vi "bats.parser.hostToFpga.testRunner.vi"(9 "Test.Messages":variant[](array[variant]), 10 "Expected OrderBook.Command[]":T1[](array[typedef]), 11 "Test.MessagesOld":T3[](array[typedef])) -> (0 "Failures.Count":i32=1, 2 "Passed":bool, 3 "OrderBook.Command[]":T1[](array[typedef]), 4 "Debug":u64[](array[numeric]) format="%.0x")   [LabVIEW 2020]
uses:
  <vilib>/rvi/interface/nirviOpenFPGA/nirviOpenFPGA.xnode
  <vilib>/rvi/interface/nirviMethod/nirviMethod.xnode
  <vilib>/rvi/interface/nirviCloseFPGA/nirviCloseFPGA.xnode
  <vilib>/rvi/errors/niLvFpgaMergeErrorWithErrorCode.vi
  <vilib>/FPGAPlugInAG/Dynamic/niLvFpga_ReadFifo_Dynamic.vi
  <vilib>/rvi/interface/nirviReadWriteControl/nirviReadWriteControl.xnode
  <vilib>/rvi/interface/Simulation/niFpgaSimulationCallBeginRW.vi
  <vilib>/rvi/errors/niLvFpgaAdjustHostInterfaceError.vi
  builds/fpganow.common/fpganow.common.host.lvlib
  NiFpgaLv.dll
  <vilib>/Utility/error.llb/Error Cluster From Error Code.vi
  fpga/bats.parser.test.vi
  <vilib>/FPGAPlugInAG/Dynamic/niLvFpga_WriteFifo_Dynamic.vi
  <vilib>/FPGAPlugInAG/Dynamic/niLvFpga_Close_Dynamic.vi
  pitch/oldMessageType.ctl
  pitch/SequencedUnitHeader/SequencedUnitHeader.Parameters.ctl
  pitch/SequencedUnitHeader/SequencedUnitHeader.lvclass
  Message.Spec.ctl
  pitch/Time/Time.Parameters.ctl
  pitch/Time/Time.lvclass
  pitch/AddOrder/AddOrderLong.Parameters.ctl
  pitch/AddOrder/AddOrderLong.lvclass
  pitch/ModifyOrder/ModifyOrderLong.Parameters.ctl
  pitch/ModifyOrder/ModifyOrderLong.lvclass
  builds/fpganow.common/orderbook.command.ctl
  builds/fpganow.common/fpganow.common.fpga.lvlib
  builds/fpganow.common/orderbook.command.type.ctl
panel:
  out "size(s)":i32
  out "Words.Out":u16[](array[numeric]) format="%.0x"
  out "Data.size":i32=16
  in  "Execute?":bool=TRUE
  out "Data":u64[](array[numeric]) format="%.0x"
  out "error out":errorcluster
  in  "error in":errorcluster
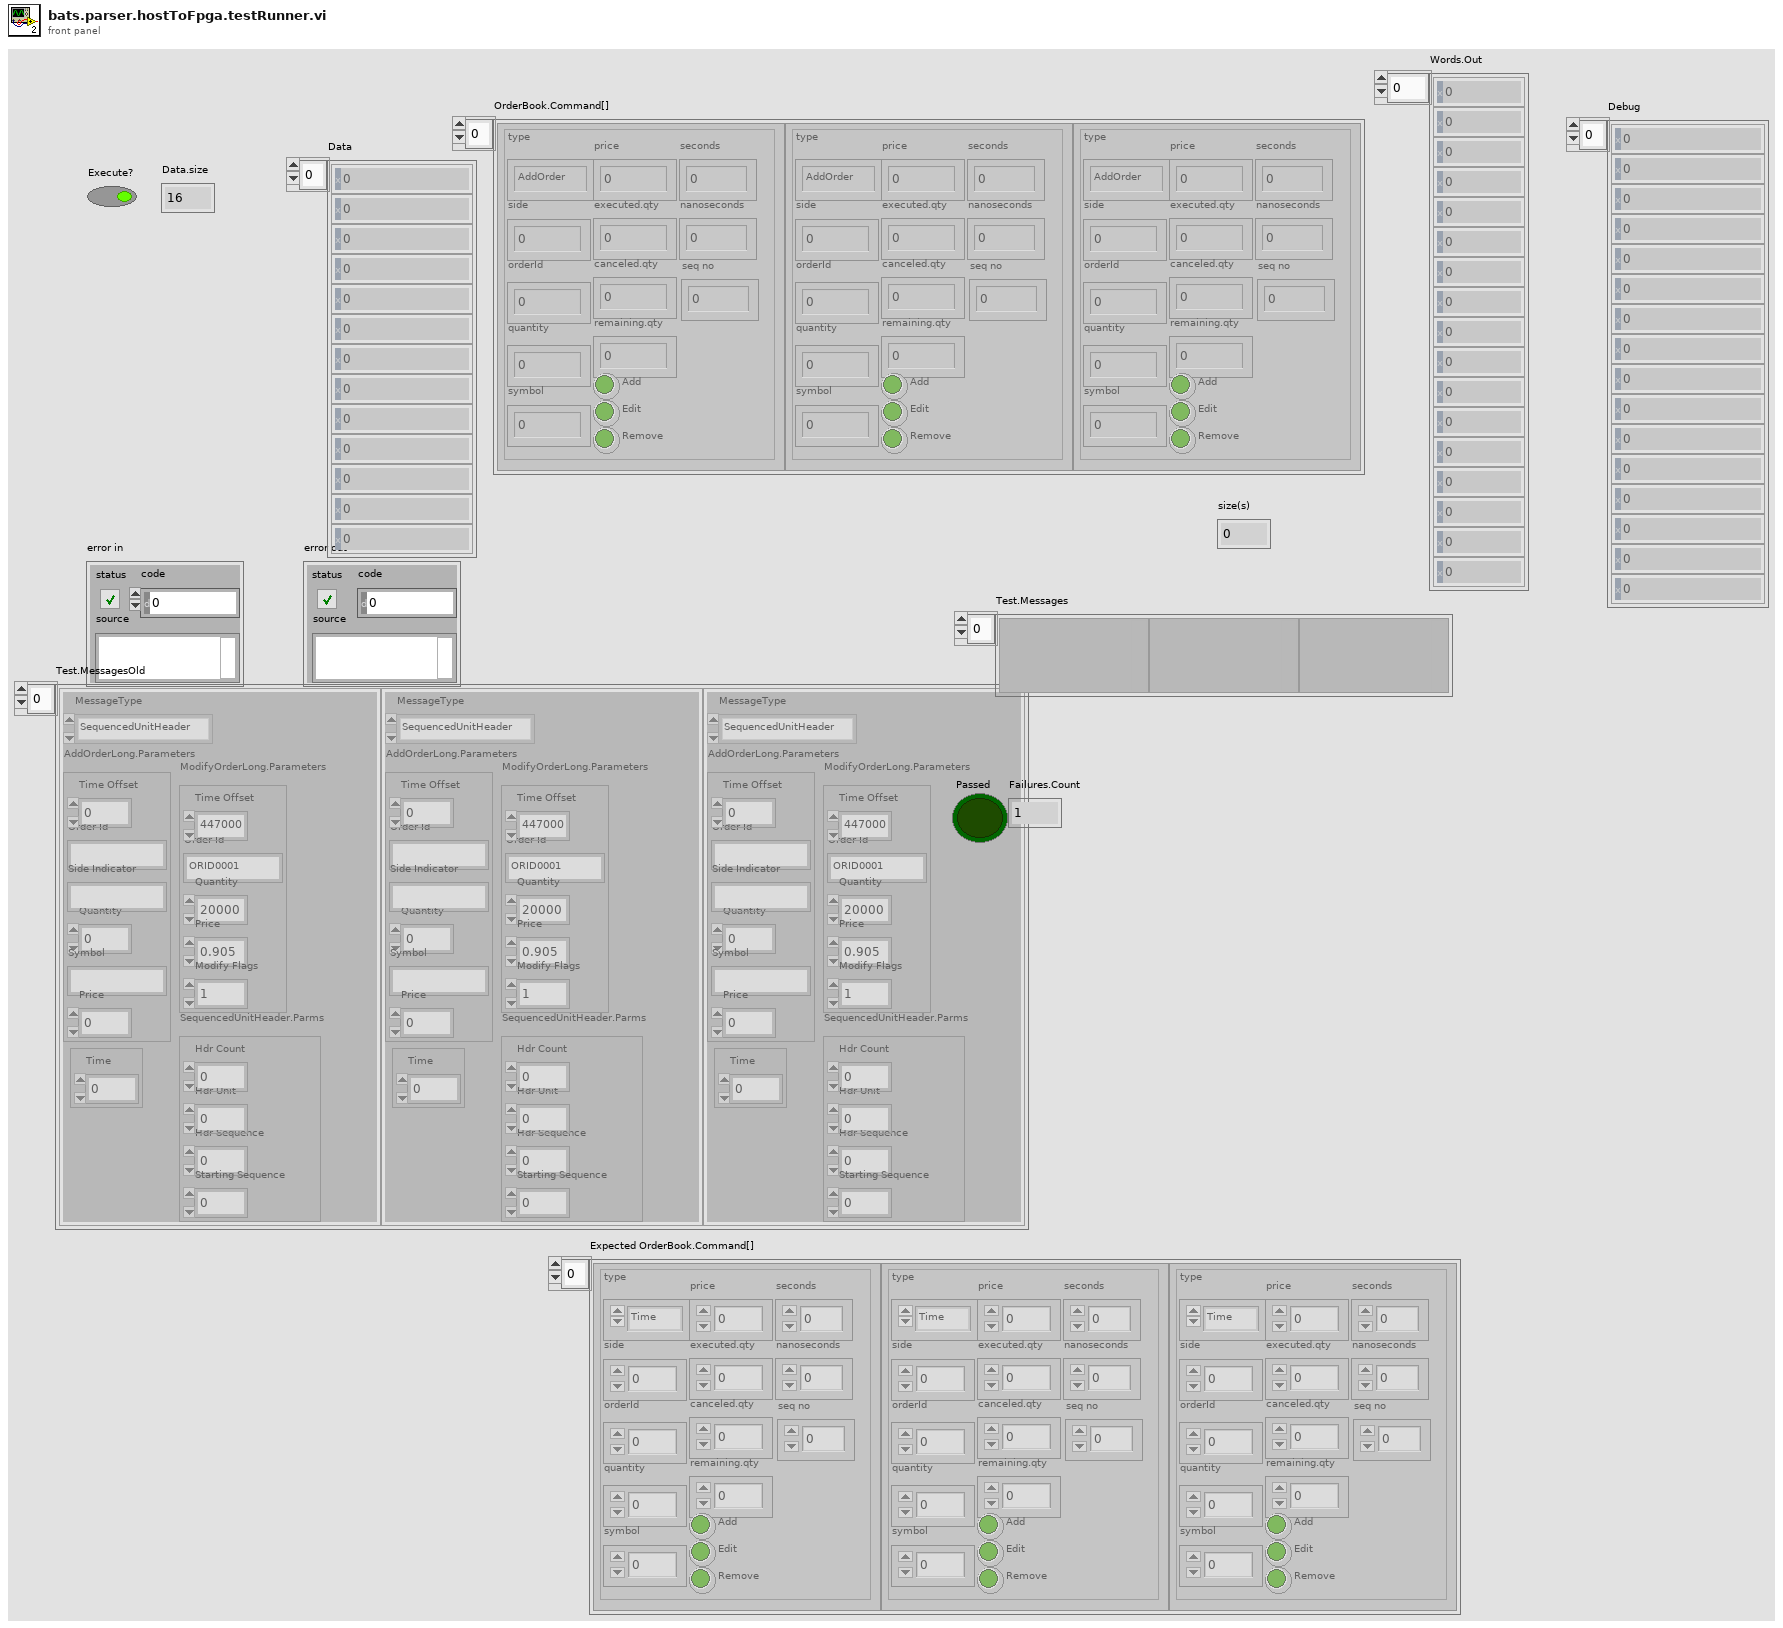
[diagram p1: front panel]
types:
  T1 = typedef "fpganow.common.fpga.lvlib/orderbook.command.ctl" = cluster{"type":T2, "side":u8, "orderId ":u64, "quantity":u32, "symbol":u64, "price":u64, "executed.qty":u32, "canceled.qty":u32, "remaining.qty":u32, "seconds":u64, "nanoseconds":u64, "Add":bool, "Edit":bool, "Remove":bool, "seq no":u32}
  T2 = typedef "fpganow.common.fpga.lvlib/orderbook.command.type.ctl" = enum8{"Time", "AddOrder", "OrderExecuted", "OrderExecutedAtPrice", "ReduceSize", "ModifyOrder", "DeleteOrder", "Get.Everything", "Get.All.Orders", "Get.Top"}
  T3 = typedef "Message.Spec.ctl" = cluster{"MessageType":T4, "AddOrderLong.Parameters":T5, "Time.Parms":T6, "SequencedUnitHeader.Parms":T7, "ModifyOrderLong.Parameters":T8}
  T4 = typedef "oldMessageType.ctl" = enum16{"Time", "SequencedUnitHeader", "AddOrderLong", "AddOrderShort", "AddOrderExpanded", "ModifyOrderLong"}
  T5 = typedef "AddOrderLong.lvclass/AddOrderLong.Parameters.ctl" = cluster{"Time Offset":u32, "Order Id":string, "Quantity":u32, "Symbol":string, "Side Indicator":string, "Price":dbl}
  T6 = typedef "Time.lvclass/Time.Parameters.ctl" = cluster{"Time":u32}
  T7 = typedef "SequencedUnitHeader.lvclass/SequencedUnitHeader.Parameters.ctl" = cluster{"Hdr Count":u8, "Hdr Unit":u8, "Hdr Sequence":u32, "Starting Sequence":u32}
  T8 = typedef "ModifyOrderLong.lvclass/ModifyOrderLong.Parameters.ctl" = cluster{"Time Offset":u32, "Order Id":string, "Quantity":u32, "Price":dbl, "Modify Flags":u8}
  T9 = cluster{"type":bool, "side":bool, "orderId ":bool, "quantity":bool, "symbol":bool, "price":bool, "executed.qty":bool, "canceled.qty":bool, "remaining.qty":bool, "seconds":bool, "nanoseconds":bool, "Add":bool, "Edit":bool, "Remove":bool, bool}
  T10 = cluster{"Index":i32, "x = y?":cluster{"type":bool, "side":bool, "orderId ":bool, "quantity":bool, "symbol":bool, "price":bool, "executed.qty":bool, "canceled.qty":bool, "remaining.qty":bool, "seconds":bool, "nanoseconds":bool, "Add":bool, "Edit":bool, "Remove":bool, bool}}
  T11 = cluster{"Index":i32, "x = y?":cluster{"type":bool, "side":bool, "orderId ":bool, "quantity":bool, "symbol":bool, "price":bool, "executed.qty":bool, "canceled.qty":bool, "remaining.qty":bool, "seconds":bool, "nanoseconds":bool, "Add":bool, "Edit":bool, "Remove":bool, bool}}[]
  T12 = cluster{"type":bool, "side":bool, "orderId ":bool, "quantity":bool, "symbol":bool, "price":bool, "executed.qty":bool, "canceled.qty":bool, "remaining.qty":bool, "seconds":bool, "nanoseconds":bool, "Add":bool, "Edit":bool, "Remove":bool, "seq no":bool}
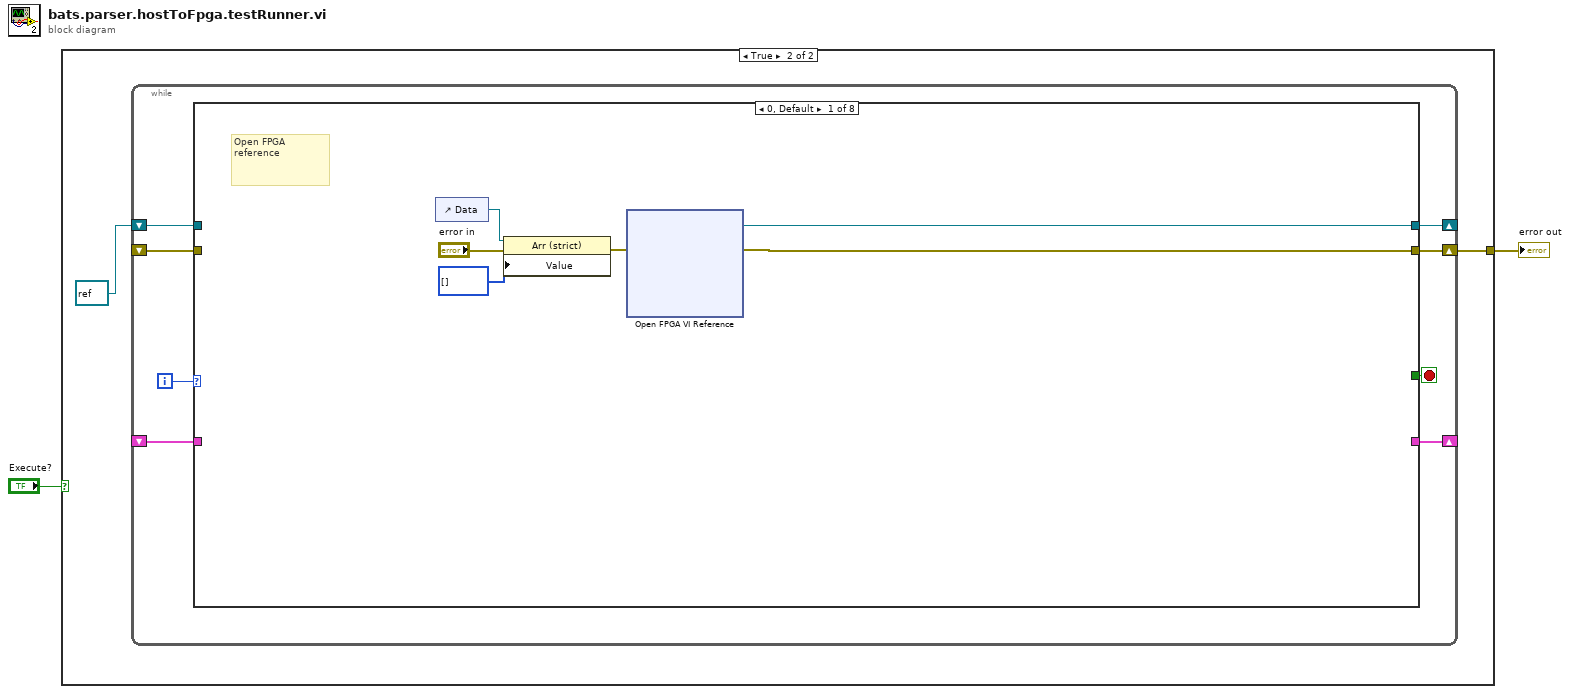
[diagram p0: block diagram]
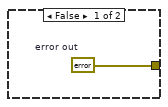
[diagram p2: hidden frame]
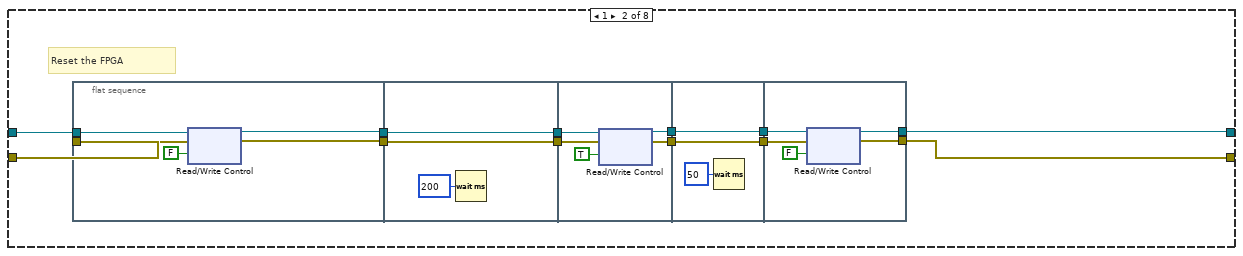
[diagram p3: hidden frame]
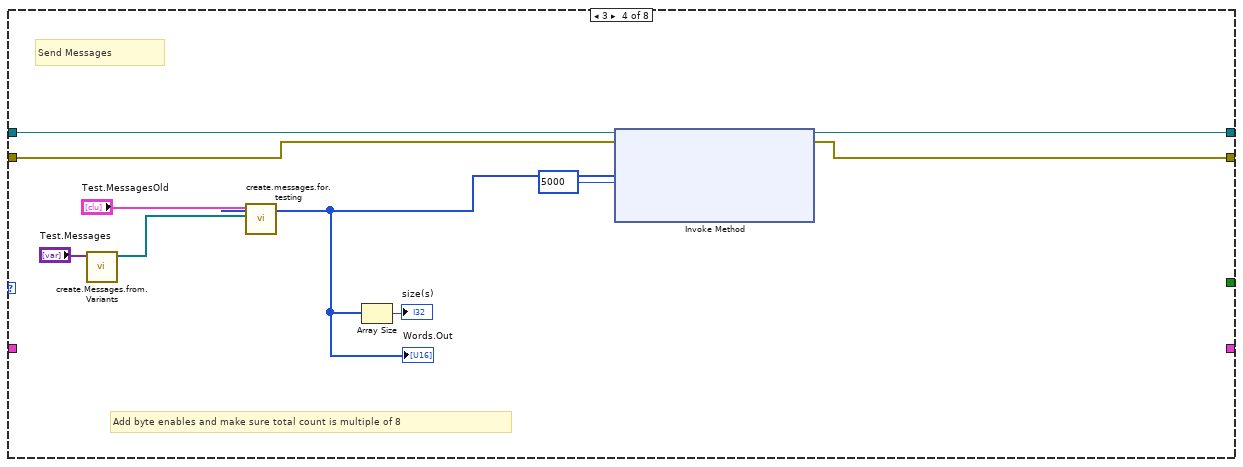
[diagram p5: hidden frame]
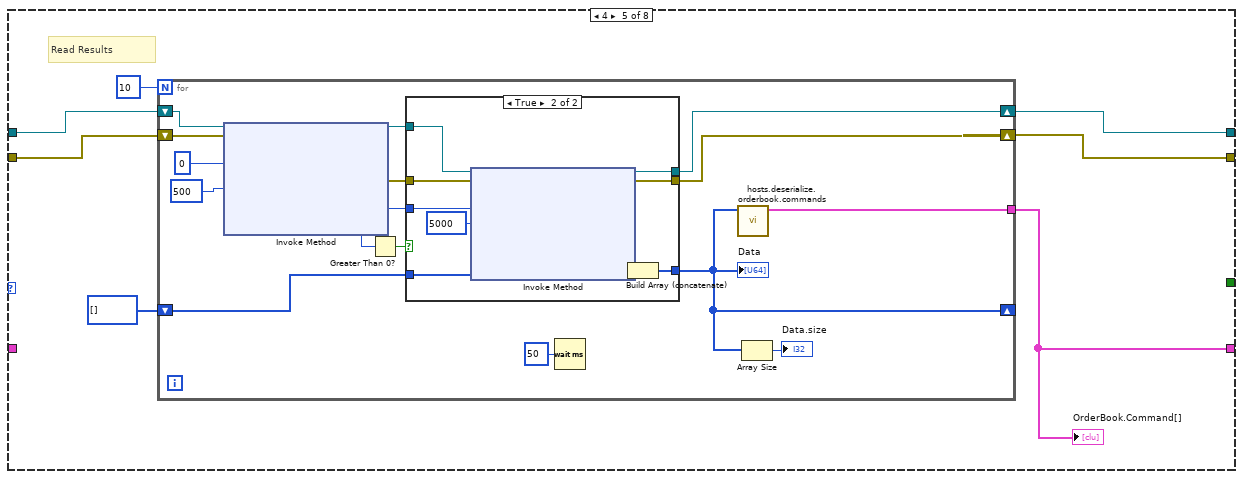
[diagram p6: hidden frame]
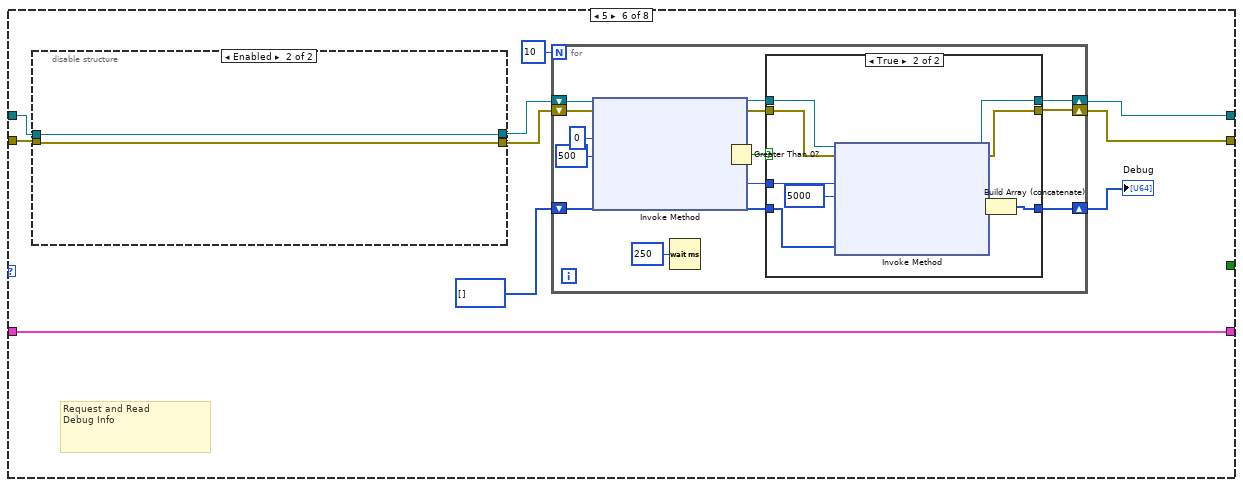
[diagram p8: hidden frame]
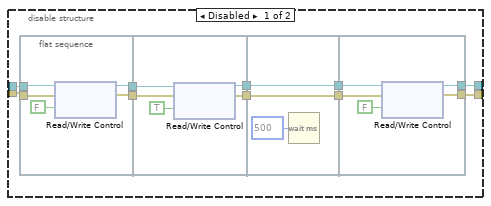
[diagram p9: hidden frame]
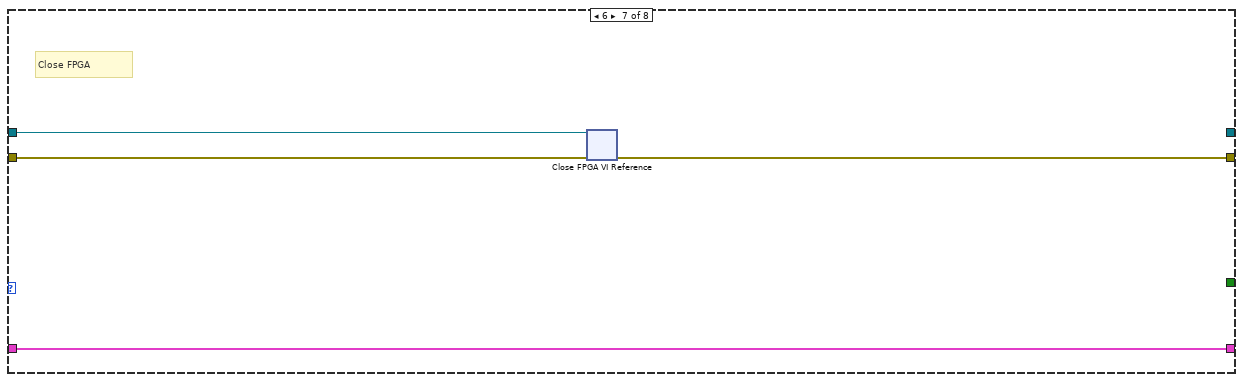
[diagram p11: hidden frame]
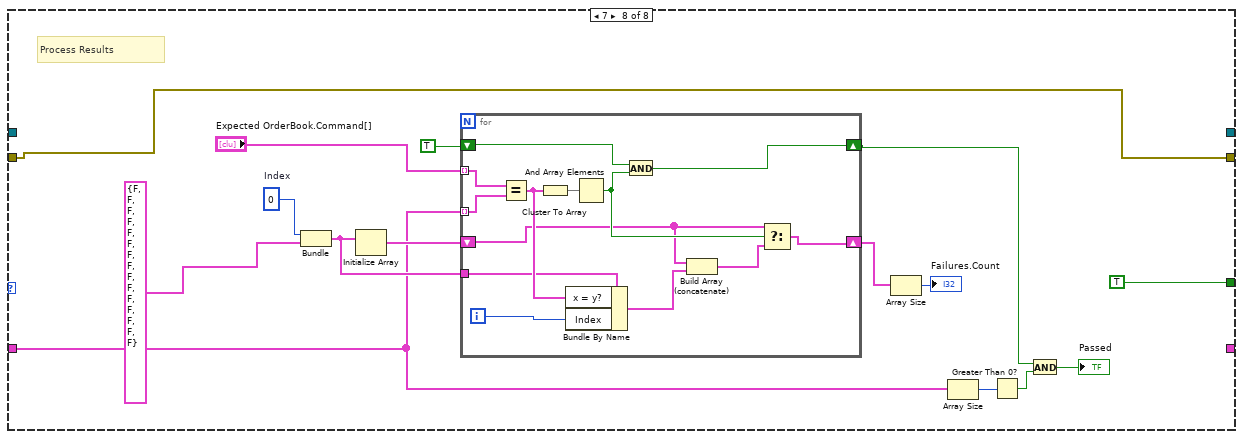
[diagram p12: hidden frame]
diagram:
  n1 = case shown="True" "Execute?" {
    tunnel: [w3 w5] -> w2
    frame False {
      w3 = errorcluster {"status"=FALSE, "code"=0, "source"=""}  # error out
    }
    frame True {
      n2 = while {
        shift-right: [w11] -> _
        shift-left: refnum<k20> refnum ("FPGA VI Reference Out") -> [w9]
        shift-right: [w10] -> w5
        shift-left: _ -> [w8]
        shift-right: [w7] -> _
        shift-left: _ -> [w6]
        i -> [w13]
        stop <- w12 stop-if-true
        n3 = case shown="0, Default" w13 {
          tunnel: [_ _ _ _ _ _ _ TRUE] -> w12
          tunnel: [w14 w24 w54 w60 w66 w103 _ _] -> w11
          tunnel: [w15 w25 w53 w59 w67 w104 w167 w169] -> w10
          tunnel: w9 -> [_ w27 w54 w62 w69 w107 w166 _]
          tunnel: w8 -> [_ w26 w53 w61 w68 w108 w165 w169]
          tunnel: [_ _ _ _ w65 w99 w164 _] -> w7
          tunnel: w6 -> [_ _ _ _ _ w99 w164 w170]
          frame 0, Default {
            # "Open FPGA\nreference"
            n4 = control-ref of="Data"() -> (w17:refnum<vi>)
            n5 = property class="Arr (strict)"(reference=w17, error in="error in", "Value"=u8[] []) -> (error out=w19:errorcluster)  [unwired: 1 out]
            n6 = xnode ("Open FPGA VI Reference")("error in"=w19) -> ("FPGA VI Reference Out"=w14:refnum<k20>, "error out"=w15:errorcluster)  [unwired: 1 in]
          }
          frame 1 {
            # "Reset the FPGA"
            n7 = flat-sequence {
              tunnel: [w35] -> w23
              tunnel: [w36] -> w21
              tunnel: w27 -> [w33]
              tunnel: w26 -> [w34]
              tunnel: w23 -> [w39]
              tunnel: [w39] -> w22
              tunnel: w21 -> [w38]
              tunnel: [w38] -> w20
              tunnel: [w43] -> w31
              tunnel: [w42] -> w30
              tunnel: w22 -> [w41]
              tunnel: w20 -> [w40]
              tunnel: [w47] -> w29
              tunnel: w31 -> [w47]
              tunnel: w30 -> [w46]
              tunnel: [w46] -> w28
              tunnel: w29 -> [w51]
              tunnel: w28 -> [w50]
              tunnel: [w49] -> w25
              tunnel: [w48] -> w24
              frame #0 {
                n8 = xnode "Read/Write Control"("FPGA VI Reference In"=w33, "error in"=w34, "reset"=FALSE) -> ("FPGA VI Reference Out"=w36:refnum<k20>, "error out"=w35:errorcluster)
              }
              frame #1 {
                n9 = Wait (ms)(milliseconds to wait=u32 200) -> ()  [unwired: 1 out]
              }
              frame #2 {
                n10 = xnode "Read/Write Control"("FPGA VI Reference In"=w40, "error in"=w41, "reset"=TRUE) -> ("FPGA VI Reference Out"=w42:refnum<k20>, "error out"=w43:errorcluster)
              }
              frame #3 {
                n11 = Wait (ms)(milliseconds to wait=u32 50) -> ()  [unwired: 1 out]
              }
              frame #4 {
                n12 = xnode "Read/Write Control"("FPGA VI Reference In"=w50, "error in"=w51, "reset"=FALSE) -> ("FPGA VI Reference Out"=w48:refnum<k20>, "error out"=w49:errorcluster)
              }
            }
          }
          frame 2 {
            # "Memory Configuration"
          }
          frame 3 {
            # "Add byte enables and make sure total count is multiple of 8"
            # "Send Messages"
            n13 = call "create.Messages.from.Variants.vi"("Messages.Variant"="Test.Messages") -> ("Messages"=w55:refnum<class "MessageBase.lvclass">[])  [unwired: 10 in]
            n14 = call "create.messages.for.testing.vi"("Message.to.Create"=w55, "Messages to Create"="Test.MessagesOld") -> ("Words.Out"=w58:u16[])  [unwired: 9 in]
            "Words.Out" <- w58
            n15 = Array Size(array=w58) -> (size(s)=→"size(s)":i32)
            n16 = xnode "Invoke Method"("FPGA VI Reference In"=w62, "error in"=w61, "Data"=w58, "Timeout (ms)"=5000) -> ("FPGA VI Reference Out"=w60:refnum<k20>, "error out"=w59:errorcluster)  [unwired: 1 out]
          }
          frame 4 {
            # "Read Results"
            n17 = for {
              N: 10 -> [_]
              shift-right: [w74] -> _
              shift-left: u64[] [] -> [w79]
              shift-right: [w78] -> w66
              shift-left: w69 -> [w86]
              shift-right: [w77] -> w67
              shift-left: w68 -> [w85]
              tunnel: [w72] -> w65
              n18 = xnode "Invoke Method"("FPGA VI Reference In"=w86, "error in"=w85, "Number of Elements"=u32 0, "Timeout (ms)"=500) -> ("FPGA VI Reference Out"=w80:refnum<k20>, "error out"=w76:errorcluster, "Elements Remaining"=w81:u32)  [unwired: 1 out]
              n19 = Greater Than 0?(x=w81) -> (x > 0?=w82:bool)
              n20 = case shown="True" w82 {
                tunnel: w81 -> [_ w98]
                tunnel: w80 -> [w88 w96]
                tunnel: [w89 w93] -> w74
                tunnel: w79 -> [w89 w95]
                tunnel: [w88 w92] -> w78
                tunnel: [w87 w91] -> w77
                tunnel: w76 -> [w87 w90]
                frame False {
                }
                frame True {
                  n21 = xnode "Invoke Method"("FPGA VI Reference In"=w96, "error in"=w90, "Number of Elements"=w98, "Timeout (ms)"=5000) -> ("FPGA VI Reference Out"=w92:refnum<k20>, "error out"=w91:errorcluster, "Data"=w94:u64[])  [unwired: 1 out]
                  n22 = Build Array (concatenate)(w95, w94) -> (w93:u64[])
                }
              }
              "Data" <- w74
              n23 = Wait (ms)(milliseconds to wait=u32 50) -> ()  [unwired: 1 out]
              n24 = call "hosts.deserialize.orderbook.commands.vi"("DataIn"=w74) -> ("OrderBook.Command[]"=w72:T1[])  [unwired: 10 in]
              n25 = Array Size(array=w74) -> (size(s)=→"Data.size":i32)
            }
            "OrderBook.Command[]" <- w65
          }
          frame 5 {
            # "Request and Read\nDebug Info"
            n26 = disable-structure shown="Enabled" {
              disable-tunnel: w108 -> [w112 w137]
              disable-tunnel: w107 -> [w111 w138]
              disable-tunnel: [w110 w138] -> w106
              disable-tunnel: [w109 w137] -> w105
              frame Disabled {
                n27 = flat-sequence {
                  tunnel: w111 -> [w120]
                  tunnel: w112 -> [w121]
                  tunnel: [w122] -> w118
                  tunnel: [w123] -> w117
                  tunnel: [w127] -> w116
                  tunnel: [w126] -> w115
                  tunnel: w118 -> [w125]
                  tunnel: w117 -> [w124]
                  tunnel: [w131] -> w114
                  tunnel: w116 -> [w131]
                  tunnel: w115 -> [w130]
                  tunnel: [w130] -> w113
                  tunnel: w114 -> [w135]
                  tunnel: w113 -> [w134]
                  tunnel: [w133] -> w109
                  tunnel: [w132] -> w110
                  frame #0 {
                    n28 = xnode "Read/Write Control"("FPGA VI Reference In"=w120, "error in"=w121, "debug"=FALSE ("reset")) -> ("FPGA VI Reference Out"=w123:refnum<k20>, "error out"=w122:errorcluster)
                  }
                  frame #1 {
                    n29 = xnode "Read/Write Control"("FPGA VI Reference In"=w124, "error in"=w125, "debug"=TRUE ("reset")) -> ("FPGA VI Reference Out"=w126:refnum<k20>, "error out"=w127:errorcluster)
                  }
                  frame #2 {
                    n30 = Wait (ms)(milliseconds to wait=u32 500) -> ()  [unwired: 1 out]
                  }
                  frame #3 {
                    n31 = xnode "Read/Write Control"("FPGA VI Reference In"=w134, "error in"=w135, "debug"=FALSE ("reset")) -> ("FPGA VI Reference Out"=w132:refnum<k20>, "error out"=w133:errorcluster)
                  }
                }
              }
              frame Enabled {
              }
            }
            n32 = for {
              N: 10 -> [_]
              shift-right: [w145] -> w103
              shift-left: w106 -> [w151]
              shift-right: [w144] -> w104
              shift-left: w105 -> [w150]
              shift-right: [w146] -> w102
              shift-left: u64[] [] -> [w140]
              n33 = xnode "Invoke Method"("FPGA VI Reference In"=w151, "error in"=w150, "Number of Elements"=u32 0, "Timeout (ms)"=500) -> ("FPGA VI Reference Out"=w143:refnum<k20>, "error out"=w142:errorcluster, "Elements Remaining"=w141:u32)  [unwired: 1 out]
              n34 = Wait (ms)(milliseconds to wait=u32 250) -> ()  [unwired: 1 out]
              n35 = Greater Than 0?(x=w141) -> (x > 0?=w147:bool)
              n36 = case shown="True" w147 {
                tunnel: [w152 w162] -> w146
                tunnel: [w154 w161] -> w145
                tunnel: [w153 w160] -> w144
                tunnel: w143 -> [w154 w159]
                tunnel: w142 -> [w153 w158]
                tunnel: w141 -> [_ w157]
                tunnel: w140 -> [w152 w155]
                frame False {
                }
                frame True {
                  n37 = xnode "Invoke Method"("FPGA VI Reference In"=w159, "error in"=w158, "Number of Elements"=w157, "Timeout (ms)"=5000) -> ("FPGA VI Reference Out"=w161:refnum<k20>, "error out"=w160:errorcluster, "Data"=w163:u64[])  [unwired: 1 out]
                  n38 = Build Array (concatenate)(w155, w163) -> (w162:u64[])
                }
              }
            }
            "Debug" <- w102
          }
          frame 6 {
            # "Close FPGA"
            n39 = xnode "Close FPGA VI Reference"("FPGA VI Reference In"=w166, "error in"=w165) -> ("error out"=w167:errorcluster)
          }
          frame 7 {
            w172 = 0  # Index
            # "Process Results"
            n40 = Bundle("Index"=w172, "x = y?"=T9 {"type"=FALSE, "side"=FALSE, "orderId "=FALSE, "quantity"=FALSE, "symbol"=FALSE, "price"=FALSE, "executed.qty"=FALSE, "canceled.qty"=FALSE, "remaining.qty"=FALSE, "seconds"=FALSE, "nanoseconds"=FALSE, "Add"=FALSE, "Edit"=FALSE, "Remove"=FALSE, FALSE}) -> (w174:T10)  [unwired: 1 in]
            n41 = Initialize Array(w174) -> (w173:T11)  [unwired: 1 in]
            n42 = for {
              tunnel: "Expected OrderBook.Command[]" -> [w195] mode=indexing
              tunnel: w170 -> [w194] mode=indexing
              shift-right: [w192] -> w181
              shift-left: TRUE -> [w193]
              shift-right: [w189] -> w175
              shift-left: w173 -> [w184]
              tunnel: w174 -> [w187]
              i -> [w186]
              n43 = Equal?(x=w195, y=w194) -> (x = y?=w188:T12)
              n44 = Cluster To Array(cluster=w188) -> (array=w191:bool[])
              n45 = Bundle By Name(cluster=w187, "x = y?"=w188, "Index"=w186) -> (w185:T10)
              n46 = And Array Elements(Boolean array=w191) -> (logical AND=w190:bool)
              n47 = And(x=w193, y=w190) -> (x .and. y?=w192:bool)
              n48 = Build Array (concatenate)(w184, w185) -> (w183:T11)
              n49 = Select(t=w184, s=w190, f=w183) -> (s? t:f=w189:T11)
            }
            n50 = Array Size(array=w175) -> (size(s)=→"Failures.Count":i32)
            n51 = Array Size(array=w170) -> (size(s)=w178:i32)
            n52 = Greater Than 0?(x=w178) -> (x > 0?=w179:bool)
            n53 = And(x=w181, y=w179) -> (x .and. y?=→"Passed":bool)
          }
        }
      }
    }
  }
  "error out" <- w2
